vi "CheckSettingsPath.vi"(11 "path (use dialog)":path=path "/Users/crogers/Documents/LabVIEW Data/ViolinCompare") -> ()   [LabVIEW 2022 SP3]
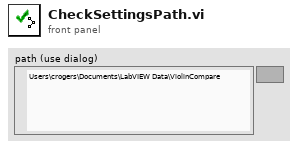
[diagram p1: front panel]
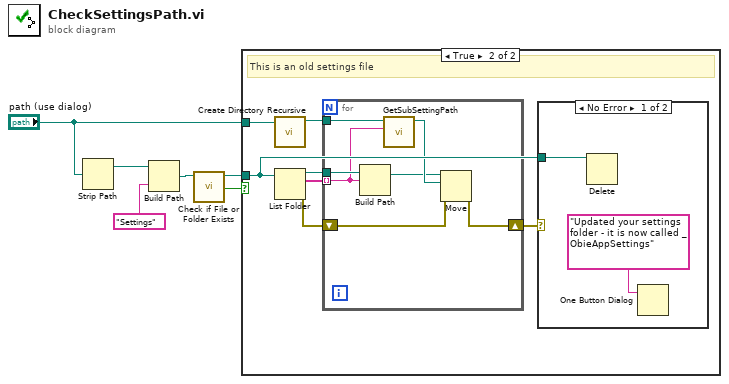
[diagram p0: block diagram]
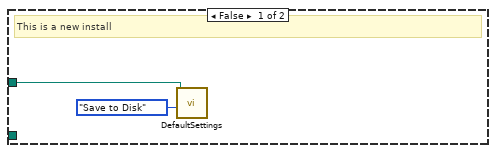
[diagram p2: hidden frame]
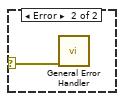
[diagram p3: hidden frame]
diagram:
  n1 = Strip Path(path="path (use dialog)") -> (stripped path=w5:path)  [unwired: 1 out]
  n2 = Build Path(base path=w5, name or relative path="Settings") -> (appended path=w6:path)
  n3 = call <vilib>:"Check if File or Folder Exists.vi"("path"=w6) -> ("file or folder exists?"=w3:bool, "dup path"=w1:path)  [unwired: 8 in, 1 out]
  n4 = case shown="True" w3 {
    tunnel: "path (use dialog)" -> [w7 w15]
    tunnel: w1 -> [_ w9]
    frame False {
      # "This is a new install"
      n5 = call "DefaultSettings.vi"("Task"=enum16{"Load to VI", "Save to Disk"}."Save to Disk", "path (use dialog)"=w7) -> ()  [unwired: 9 in, 1 out]
    }
    frame True {
      # "This is an old settings file"
      n6 = call <vilib>:"Create Directory Recursive.vi"("directory"=w15) -> ("directory copy"=w11:path)  [unwired: 4 in, 2 out]
      n7 = List Folder(path=w9) -> (path out=w13:path, filenames=w12:string[], error out=w14:errorcluster)  [unwired: 3 in, 1 out]
      n8 = for {
        tunnel: w13 -> [w24]
        tunnel: w12 -> [w22] mode=indexing
        tunnel: w11 -> [w23]
        shift-right: [w19] -> w10
        shift-left: w14 -> [w25]
        n9 = Build Path(base path=w24, name or relative path=w22) -> (appended path=w20:path)
        n10 = call "GetSubSettingPath.vi"("settings file name"=w22, "LabVIEW Data Path"=w23) -> ("settings file path"=w21:path)  [unwired: 9 in]
        n11 = Move(source path=w20, error in=w25, 10:w21) -> (error out=w19:errorcluster)  [unwired: 2 in, 2 out]
      }
      n12 = case shown="No Error" w10 {
        selector: w10 -> [_ w18]
        tunnel: w9 -> [w16 _]
        frame No Error {
          n13 = Delete(path (use dialog)=w16) -> ()  [unwired: 4 in, 3 out]
          n14 = One Button Dialog(message="Updated your settings folder - it is now called _ObieAppSettings" ("name or relative path")) -> ()  [unwired: 1 in, 1 out]
        }
        frame Error {
          n15 = call <vilib>:"General Error Handler.vi"("error in (no error)"=w18) -> ()  [unwired: 10 in, 5 out]
        }
      }
    }
  }
